vi "PXI-2510 Initialization VI.vi"(8 "error in (no error)":errorcluster, 10 "Custom XML":string, 11 "Device Item Ref in":T3 format="%.0x") -> (0 "error out":errorcluster, 3 "Device Item Ref out":T3 format="%.0x")   [LabVIEW 2011, in "PXI-2510 Custom Device.lvlib"]
uses:
  PXI-2510 Custom Device.lvlib
  <vilib>/NI Veristand/Custom Device API/Custom Device Item Ref.ctl
  <vilib>/NI Veristand/Custom Device API/Custom Device Channel.ctl
  <vilib>/NI Veristand/Custom Device API/Custom Device Channel Type.ctl
  <vilib>/NI Veristand/Custom Device API/Custom Device Timed Loop Priority.ctl
  <vilib>/NI Veristand/Custom Device API/Custom Device Loop Type.ctl
  Fault Bus Input Selector.ctl
  FIU Global Strings.vi
  <vilib>/NI Veristand/Custom Device API/Custom Device API.lvlib
panel:
  in  "Channel":T1
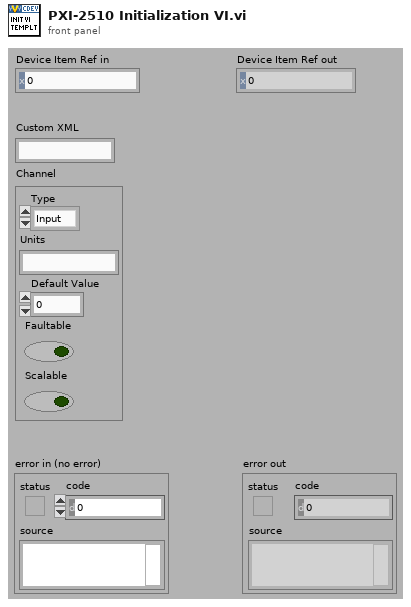
[diagram p1: front panel]
types:
  T1 = typedef "Custom Device API.lvlib/Custom Device Channel.ctl" = cluster{"Type":T2, "Units":string, "Default Value":dbl, "Faultable":bool, "Scalable":bool}
  T2 = typedef "Custom Device API.lvlib/Custom Device Channel Type.ctl" = enum16{"Input", "Output"}
  T3 = typedef "Custom Device API.lvlib/Custom Device Item Ref.ctl" = u64
  T4 = typedef "Custom Device API.lvlib/Custom Device Timed Loop Priority.ctl" = enum32{"Low", "Medium", "High"}
  T5 = typedef "Custom Device API.lvlib/Custom Device Loop Type.ctl" = enum32{"While Loop", "Timed Loop"}
  T6 = typedef "PXI-2510 Custom Device.lvlib/Fault Bus Input Selector.ctl" = enum16{"Default", "Input 0", "Input 1", "Input 2", "Input 3", "Main Bus Only"}
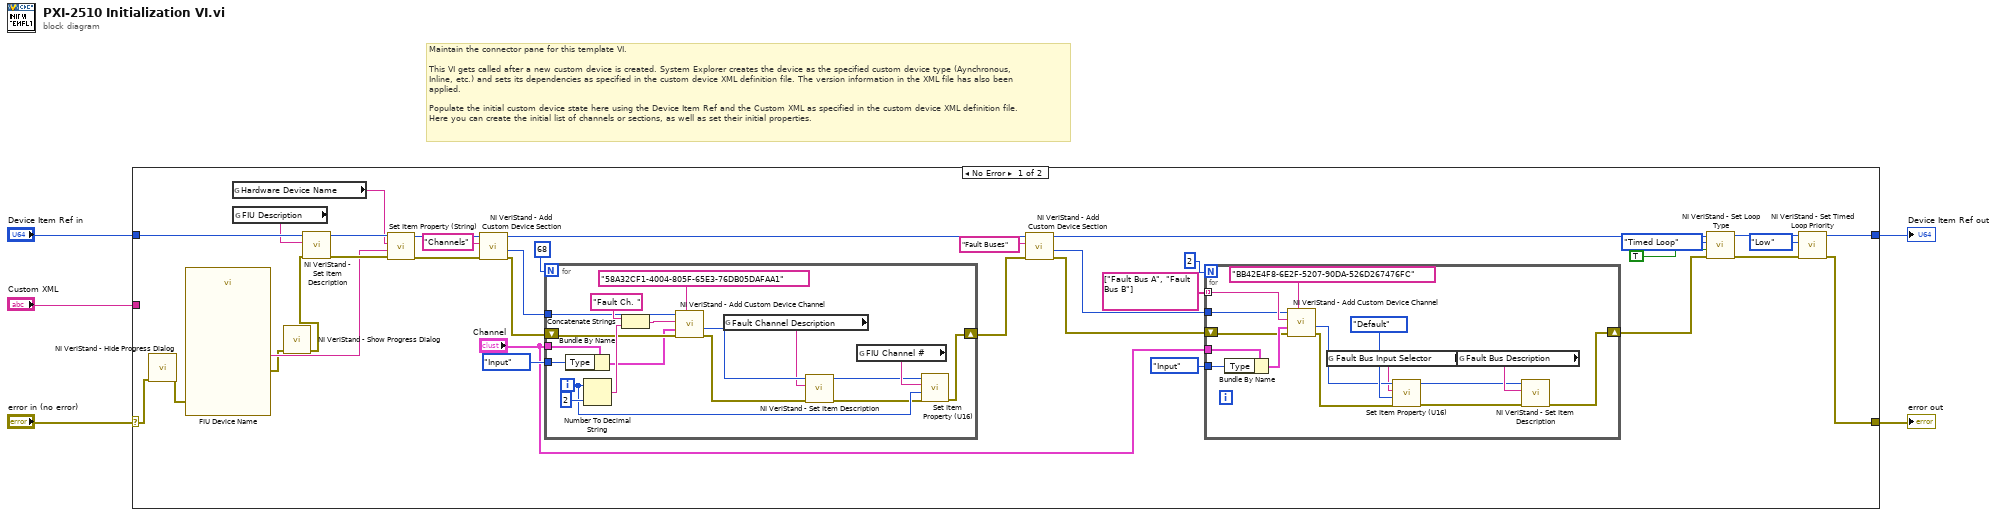
[diagram p0: block diagram]
diagram:
  # "Maintain the connector pane for this template VI.\n\nThis VI gets called after a new custom device is created. System Explorer creates the device as the specified custom device type (Aynchronous, Inline, etc.) and sets its dependencies as specified in the custom device XML definition file. The version information in the XML file has also been applied.\n\nPopulate the initial custom device state here using the Device Item Ref and the Custom XML as specified in the custom device XML definition file. Here you can create the initial list of channels or sections, as well as set their initial properties."
  n1 = case shown="No Error" "error in (no error)" {
    selector: "error in (no error)" -> [w8 w75]
    tunnel: [w13 w75] -> w5
    tunnel: [w14 w74] -> w3
    tunnel: "Device Item Ref in" -> [w40 w74]
    tunnel: "Custom XML" -> [_ _]
    frame No Error {
      n2 = call <vilib>:"NI VeriStand - Hide Progress Dialog.vi"("error in (no error)"=w8) -> ("error out"=w9:errorcluster)  [unwired: 10 in]
      n3 = call "FIU Device Name"("error in (no error)"=w9) -> ("MAX Device Name"=w10:string, "error out"=w7:errorcluster)  [unwired: 16 in, 1 out]
      n4 = global read "FIU Global Strings.vi" "Hardware Device Name"() -> (w15:string)
      n5 = global read "FIU Global Strings.vi" "FIU Description"() -> (w32:string)
      n6 = call <vilib>:"NI VeriStand - Show Progress Dialog.vi"("error in (no error)"=w7) -> ("error out"=w6:errorcluster)  [unwired: 10 in]
      n7 = call <vilib>:"NI VeriStand - Set Item Description.vi"("error in (no error)"=w6, "Description"=w32, "Item Ref in"=w40) -> ("error out"=w34:errorcluster, "Item Ref out"=w33:T3)  [unwired: 6 in, 1 out]
      n8 = call <vilib>:"Set Item Property (String).vi"("error in (no error)"=w34, "Value"=w10, "Property Name"=w15, "Item Ref in"=w33) -> ("error out"=w30:errorcluster, "Item Ref out"=w21:T3)  [unwired: 5 in, 1 out]
      n9 = call <vilib>:"NI VeriStand - Add Custom Device Section.vi"("error in (no error)"=w30, "Section Name"="Channels", "Parent Ref in"=w21) -> ("error out"=w28:errorcluster, "Section Ptr"=w17:T3, "Parent Ref out"=w19:T3)  [unwired: 5 in, 1 out]
      n10 = for {
        N: 68 -> [_]
        tunnel: "Channel" -> [w72]
        tunnel: Custom_Device_Channel_Type."Input" ("Type") -> [w68]
        shift-right: [w61] -> w23
        shift-left: w28 -> [w67]
        tunnel: w17 -> [w65]
        i -> [w63]
        n11 = Bundle By Name(cluster=w72, "Type"=w68) -> (w66:T1)
        n12 = Number To Decimal String(number=w63, width (-)=i16 2) -> (decimal integer string=w70:string)
        n13 = Concatenate Strings("Fault Ch. " ("Section Name"), w70) -> (w69:string)
        n14 = call <vilib>:"NI VeriStand - Add Custom Device Channel.vi"("GUID (Default Channel)"="58A32CF1-4004-805F-65E3-76DB05DAFAA1", "error in (no error)"=w67, "Channel"=w66, "Channel Name"=w69, "Parent Ref in"=w65) -> ("error out"=w58:errorcluster, "Channel Ref"=w60:T3)  [unwired: 3 in, 2 out]
        n15 = global read "FIU Global Strings.vi" "Fault Channel Description"() -> (w56:string)
        n16 = call <vilib>:"NI VeriStand - Set Item Description.vi"("error in (no error)"=w58, "Description"=w56, "Item Ref in"=w60) -> ("error out"=w57:errorcluster, "Item Ref out"=w59:T3)  [unwired: 6 in, 1 out]
        n17 = global read "FIU Global Strings.vi" "FIU Channel #"() -> (w64:string)
        n18 = call <vilib>:"Set Item Property (U16).vi"("error in (no error)"=w57, "Value"=w63, "Property Name"=w64, "Item Ref in"=w59) -> ("error out"=w61:errorcluster)  [unwired: 5 in, 2 out]
      }
      n19 = call <vilib>:"NI VeriStand - Add Custom Device Section.vi"("error in (no error)"=w23, "Section Name"="Fault Buses", "Parent Ref in"=w19) -> ("error out"=w18:errorcluster, "Section Ptr"=w16:T3, "Parent Ref out"=w12:T3)  [unwired: 5 in, 1 out]
      n20 = for {
        N: 2 -> [_]
        tunnel: "Channel" -> [w55]
        tunnel: Custom_Device_Channel_Type."Input" ("Type") -> [w53]
        shift-right: [w41] -> w11
        shift-left: w18 -> [w52]
        tunnel: string[] ["Fault Bus A", "Fault Bus B"] -> [w50] mode=indexing
        tunnel: w16 -> [w47]
        n21 = Bundle By Name(cluster=w55, "Type"=w53) -> (w54:T1)
        n22 = call <vilib>:"NI VeriStand - Add Custom Device Channel.vi"("GUID (Default Channel)"="BB42E4F8-6E2F-5207-90DA-526D267476FC", "error in (no error)"=w52, "Channel"=w54, "Channel Name"=w50, "Parent Ref in"=w47) -> ("error out"=w51:errorcluster, "Channel Ref"=w46:T3)  [unwired: 3 in, 2 out]
        n23 = global read "FIU Global Strings.vi" "Fault Bus Input Selector"() -> (w45:string)
        n24 = call <vilib>:"Set Item Property (U16).vi"("error in (no error)"=w51, "Value"=Fault_Bus_Input_Selector."Default" ("Fault Bus Input Selector"), "Property Name"=w45, "Item Ref in"=w46) -> ("error out"=w42:errorcluster, "Item Ref out"=w43:T3)  [unwired: 5 in, 1 out]
        n25 = global read "FIU Global Strings.vi" "Fault Bus Description"() -> (w44:string)
        n26 = call <vilib>:"NI VeriStand - Set Item Description.vi"("error in (no error)"=w42, "Description"=w44, "Item Ref in"=w43) -> ("error out"=w41:errorcluster)  [unwired: 6 in, 2 out]
      }
      n27 = call <vilib>:"NI VeriStand - Set Loop Type.vi"("error in (no error)"=w11, "Use Device Clock (Timed Loops only)"=TRUE, "Loop type"=Custom_Device_Loop_Type."Timed Loop", "Device Ref in"=w12) -> ("error out"=w35:errorcluster, "Device Ref out"=w36:T3)  [unwired: 6 in]
      n28 = call <vilib>:"NI VeriStand - Set Timed Loop Priority.vi"("error in (no error)"=w35, "Priority"=Custom_Device_Timed_Loop_Priority."Low", "Device Ref in"=w36) -> ("error out"=w13:errorcluster, "Device Ref out"=w14:T3)  [unwired: 7 in]
    }
    frame Error {
    }
  }
  "error out" <- w5
  "Device Item Ref out" <- w3
